vi "test_strain_mapping.vi"() -> ()   [LabVIEW 2013]
panel:
  in  "input":dbl
  in  "y":dbl[](array[numeric])=[0.0, 260.0, 512.0, 1042.0, 1395.0, 2090.0]
  in  "x":dbl[](array[numeric])=[0.0, 0.000144, 0.000283, 0.000557, 0.000751, 0.001057]
  out "out":dbl[](array[numeric])=[15.0, 25.0, 50.0]
  in  "data":dbl[](array[numeric])=[1.5, 2.5, 6.0]
  in  "input cal X":dbl[](array[numeric])=[0.0, 1.0, 2.0, 3.0, 4.0, 5.0]
  in  "output cal Y":dbl[](array[numeric])=[0.0, 10.0, 20.0, 30.0, 40.0, 50.0]
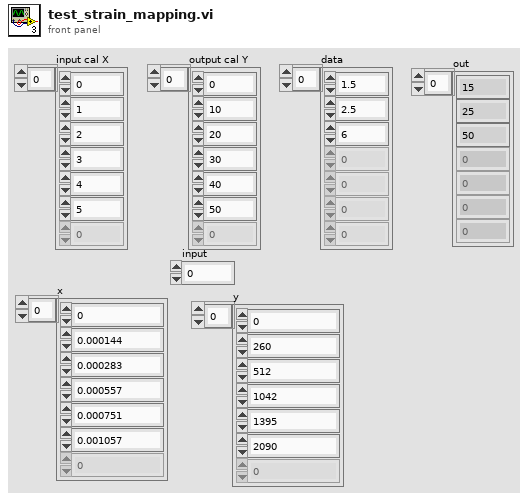
[diagram p1: front panel]
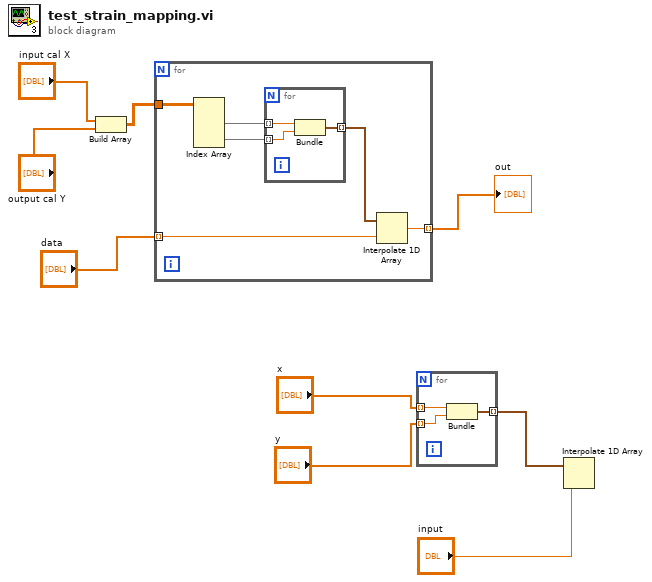
[diagram p0: block diagram]
diagram:
  n1 = Build Array("input cal X", "output cal Y") -> (w9:dbl[][])
  n2 = for {
    tunnel: w9 -> [w11]
    tunnel: [w13] -> w5 mode=indexing
    tunnel: "data" -> [w12] mode=indexing
    n3 = Index Array(array=w11) -> (element #1=w15:dbl[], element #2=w14:dbl[])  [unwired: 4 in]
    n4 = for {
      tunnel: w15 -> [w18] mode=indexing
      tunnel: w14 -> [w17] mode=indexing
      tunnel: [w16] -> w10 mode=indexing
      n5 = Bundle(w18, w17) -> (w16:cluster{dbl, dbl})  [unwired: 1 in]
    }
    n6 = Interpolate 1D Array(1:w12, 2:w10) -> (0:w13:dbl)
  }
  "out" <- w5
  n7 = for {
    tunnel: "x" -> [w21] mode=indexing
    tunnel: "y" -> [w20] mode=indexing
    tunnel: [w19] -> w2 mode=indexing
    n8 = Bundle(w21, w20) -> (w19:cluster{dbl, dbl})  [unwired: 1 in]
  }
  n9 = Interpolate 1D Array(1:"input", 2:w2) -> ()  [unwired: 1 out]
